vi "Run Test.vi"(9 "Solver Ref":refnum<vi>, 10 "Random Words Count":i32, 11 "Single Word":string) -> (0 "error out":errorcluster, 2 "Results":string, 3 "Avg Guesses":dbl=10.0, 5 "Min Guesses":i32, 7 "Max Guesses":i32)   [LabVIEW 2020, in "Wordle Engine.lvlib"]
uses:
  Wordle Engine.lvlib
  1d140959-14b4-459d-b57b-f388c12a8cde.vi
panel:
  out "Current Solve":i32
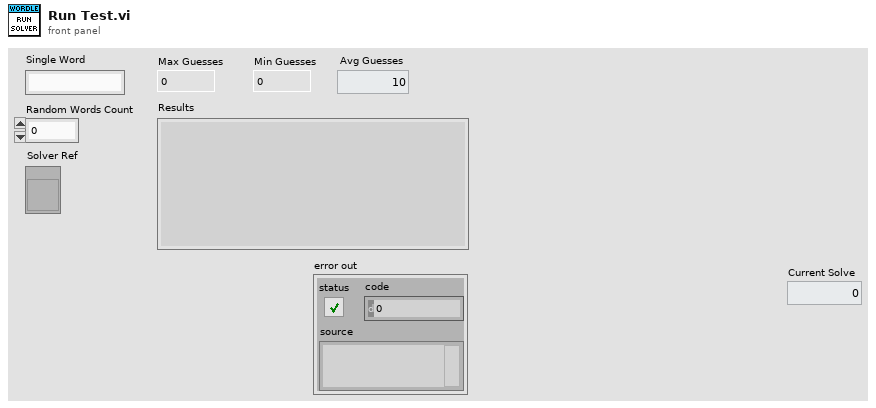
[diagram p1: front panel]
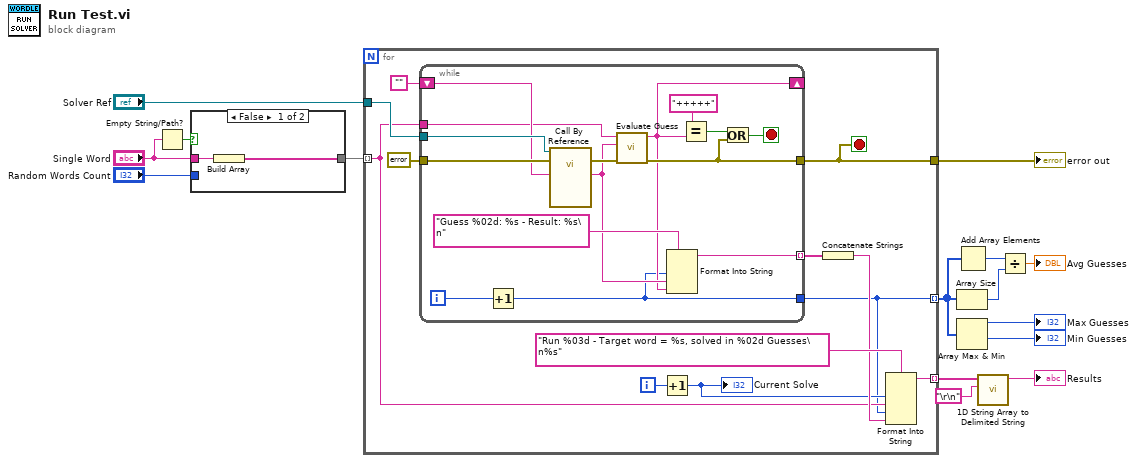
[diagram p0: block diagram]
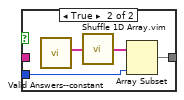
[diagram p2: hidden frame]
diagram:
  n1 = Empty String/Path?(string/path="Single Word") -> (empty?=w15:bool)
  n2 = case shown="False" w15 {
    tunnel: "Single Word" -> [w17 _]
    tunnel: "Random Words Count" -> [_ w19]
    tunnel: [w16 w18] -> w12
    frame False {
      n3 = Build Array(w17) -> (w16:string[])
    }
    frame True {
      n4 = call "Valid Answers--constant.vi"() -> ("Valid Answers Array"=w21:string[])  [unwired: 10 in, 1 out]
      n5 = call "Shuffle 1D Array.vim"("array"=w21) -> ("shuffled array"=w20:string[])  [unwired: 4 in]
      n6 = Array Subset(array=w20, length=w19) -> (w18:string[])  [unwired: 1 in]
    }
  }
  n7 = for {
    tunnel: w12 -> [w25] mode=indexing
    tunnel: "Solver Ref" -> [w33]
    tunnel: [w24] -> w4 mode=indexing
    tunnel: [w23] -> w10 mode=indexing
    tunnel: [w22] -> w1
    i -> [w26]
    stop <- w22 stop-if-true
    n8 = while {
      tunnel: w33 -> [w48]
      tunnel: errorcluster {"status"=FALSE, "code"=0, "source"=""} ("error out") -> [w47]
      tunnel: [w42] -> w22
      shift-right: [w37] -> _
      shift-left: "" -> [w46]
      tunnel: w25 -> [w45]
      tunnel: [w36] -> w27 mode=indexing
      tunnel: [w34] -> w24
      i -> [w35]
      stop <- w43 stop-if-true
      n9 = Increment(x=w35) -> (x+1=w34:i32)
      n10 = call-by-ref "?"(reference=w48, error in=w47, "Previous Guess Result"=w46) -> (error out=w44:errorcluster, "New Guess"=w38:string)  [unwired: 10 in, 1 out]
      n11 = call "Evaluate Guess.vi"("error in"=w44, "Guess"=w38, "Current Word"=w45) -> ("error out"=w42:errorcluster, "Result"=w37:string)  [unwired: 7 in]
      n12 = Format Into String(format string="Guess %02d: %s - Result: %s\n", w34, w38, w37) -> (resulting string=w36:string)  [unwired: 2 in, 1 out]
      n13 = Equal?(x="+++++", y=w37) -> (x = y?=w40:bool)
      n14 = Or(x=w40, y=w42) -> (x .or. y?=w43:bool)
    }
    n15 = Increment(x=w26) -> (x+1=w28:i32)
    "Current Solve" <- w28
    n16 = Concatenate Strings(w27) -> (w29:string)
    n17 = Format Into String(format string="Run %03d - Target word = %s, solved in %02d Guesses\n%s", w28, w25, w24, w29) -> (resulting string=w23:string)  [unwired: 2 in, 1 out]
  }
  "error out" <- w1
  n18 = Array Size(array=w4) -> (size(s)=w6:i32)
  n19 = Array Max & Min(array=w4) -> (max value=→"Max Guesses":i32, min value=→"Min Guesses":i32)  [unwired: 2 out]
  n20 = Add Array Elements(numeric array=w4) -> (sum=w7:i32)
  n21 = call <vilib>:"1D String Array to Delimited String.vi"("delimiter"="\r\n", "string array"=w10) -> ("delimited string"=→"Results":string)  [unwired: 9 in]
  n22 = Divide(x=w7, y=w6) -> (x/y=→"Avg Guesses":dbl)
